vi "Valhalla Resistance Measurement.vi"(8 "error in (no error)":errorcluster, 11 "VISA Refnum in":refnum<visa-resource-name>) -> (0 "error out":errorcluster, 1 "In Range?":bool, 2 "Current Range":string, 3 "VISA Refnum out":refnum<visa-resource-name>, 5 "Resistance":string)   [LabVIEW 2018]
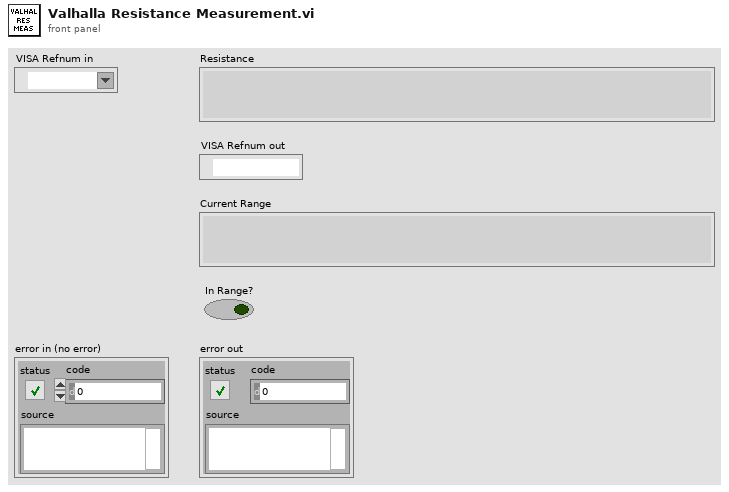
[diagram p1: front panel]
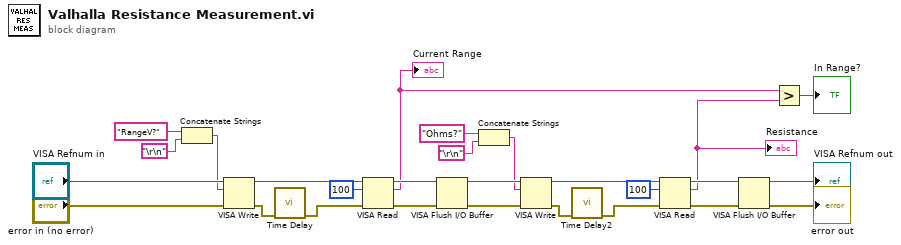
[diagram p0: block diagram]
diagram:
  n1 = Concatenate Strings("RangeV?" ("write buffer"), "\r\n") -> (w2:string)
  n2 = VISA Write(VISA resource name="VISA Refnum in", write buffer=w2, error in (no error)="error in (no error)") -> (VISA resource name out=w4:refnum<visa-resource-name>, error out=w6:errorcluster)  [unwired: 1 out]
  n3 = call "Time Delay"("error in (no error)"=w6) -> ("error out"=w5:errorcluster)  [unwired: 10 in]
  n4 = VISA Read(VISA resource name=w4, byte count=u32 100, error in (no error)=w5) -> (VISA resource name out=w22:refnum<visa-resource-name>, read buffer=w15:string, error out=w24:errorcluster)  [unwired: 1 out]
  "Current Range" <- w15
  n5 = VISA Flush I/O Buffer(VISA resource name=w22, error in (no error)=w24) -> (VISA resource name out=w23:refnum<visa-resource-name>, error out=w25:errorcluster)  [unwired: 1 in]
  n6 = Concatenate Strings("Ohms?" ("write buffer"), "\r\n") -> (w9:string)
  n7 = VISA Write(VISA resource name=w23, write buffer=w9, error in (no error)=w25) -> (VISA resource name out=w11:refnum<visa-resource-name>, error out=w13:errorcluster)  [unwired: 1 out]
  n8 = call "Time Delay2"("error in (no error)"=w13) -> ("error out"=w12:errorcluster)  [unwired: 10 in]
  n9 = VISA Read(VISA resource name=w11, byte count=u32 100, error in (no error)=w12) -> (VISA resource name out=w19:refnum<visa-resource-name>, read buffer=w16:string, error out=w18:errorcluster)  [unwired: 1 out]
  "Resistance" <- w16
  n10 = VISA Flush I/O Buffer(VISA resource name=w19, error in (no error)=w18) -> (VISA resource name out=→"VISA Refnum out":refnum<visa-resource-name>, error out=→"error out":errorcluster)  [unwired: 1 in]
  n11 = Greater?(x=w15, y=w16) -> (0:→"In Range?":bool)
